vi "Seguidor Top Level.vi"() -> ()   [LabVIEW 2017]
uses:
  <vilib>/myRIO/Instrument Drivers/Onboard IO/I2C/typedefs/I2C User Configuration.ctl
  <vilib>/myRIO/Instrument Drivers/Onboard IO/I2C/typedefs/I2C Transfer Rate.ctl
  <vilib>/myRIO/Common/Instrument Driver Framework/myRIO v1.0/UART/vis/myRIO v1.0 Close UART.vi
  <vilib>/Utility/error.llb/Error Cluster From Error Code.vi
  <vilib>/myRIO/Common/Instrument Driver Framework/myRIO v1.0/I2C/vis/myRIO v1.0 Configure I2C.vi
  <vilib>/myRIO/Common/Instrument Driver Framework/Utilities/vis/FPGA Ref Manager.vi
  <vilib>/myRIO/Common/Instrument Driver Framework/myRIO v1.0/myRIO v1.0 Reset FPGA.vi
  <vilib>/myRIO/Common/Instrument Driver Framework/myRIO v1.0/IRQ/vis/myRIO v1.0 IRQ Info FGV.vi
  <vilib>/myRIO/Common/Instrument Driver Framework/myRIO v1.0/IRQ/vis/myRIO v1.0 Timer IRQ Info FGV.vi
  <vilib>/myRIO/Common/Instrument Driver Framework/myRIO v1.0/IRQ/vis/myRIO v1.0 ISR Agent.vi
  <vilib>/myRIO/Instrument Drivers/Onboard IO/I2C/I2C.lvlib
  <vilib>/myRIO/Instrument Drivers/Utilities/Utilities.lvlib
panel:
  in  "Boolean":bool
  in  "Enum":T1(ring)
  in  "stop":bool
  in  "Adelante/Atras":bool
  in  "Motor2":enum16{"MotorB", "MotorA"}(ring)
  in  "Motor1":enum16{"MotorB", "MotorA"}(ring)
  out "White":u8
  in  "Offset":dbl
  in  "Potencia \nmotores (%)":dbl(slide) scale=-100.0..100.0
  in  "Constante de \nProporcionalidad":dbl
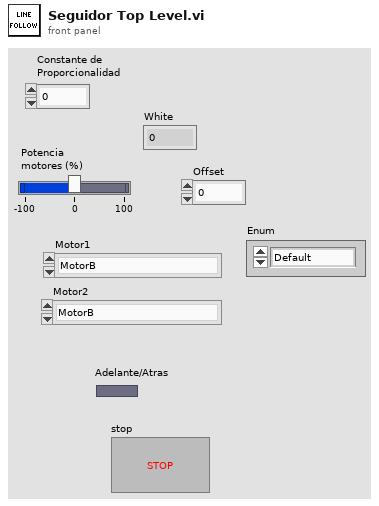
[diagram p1: front panel]
types:
  T1 = enum16{"Default", "Intersection", "Degrees", "Vision"}
  T2 = typedef "I2C.lvlib/I2C User Configuration.ctl" = cluster{"I2C Transfer Rate":T3}
  T3 = typedef "I2C.lvlib/I2C Transfer Rate.ctl" = enum16{"Standard mode (100 kbps)", "Fast mode (400 kbps)"}
  T4 = typedef "I2C.lvlib/I2C Reference.ctl" = cluster{"myRIO Reference":T5, "I2C Channels Enum":T9, "I2C Configuration":T10}
  T5 = typedef "myRIO Generic Hardware Reference.ctl" = cluster{"myRIO Model":T6, "myRIO Hardware Reference":T7}
  T6 = typedef "Hardware Version Enum.ctl" = enum16{"Unknown", "myRIO-1900", "myRIO-1950", "roboRIO", "NI ELVIS RIO CM"}
  T7 = typedef "myRIO v1.0 Reference.ctl" = cluster{"Generic FPGA Reference":T8, "Allow multiple opens":bool}
  T8 = typedef "Generic FPGA Reference.ctl" = refnum<k20>
  T9 = typedef "I2C Channels Enum.ctl" = enum16{"Not Connected", "A/I2C", "B/I2C", "I2C/I2C"}
  T10 = typedef "I2C.lvlib/I2C Configuration.ctl" = cluster{"I2C Transfer Rate":T3}
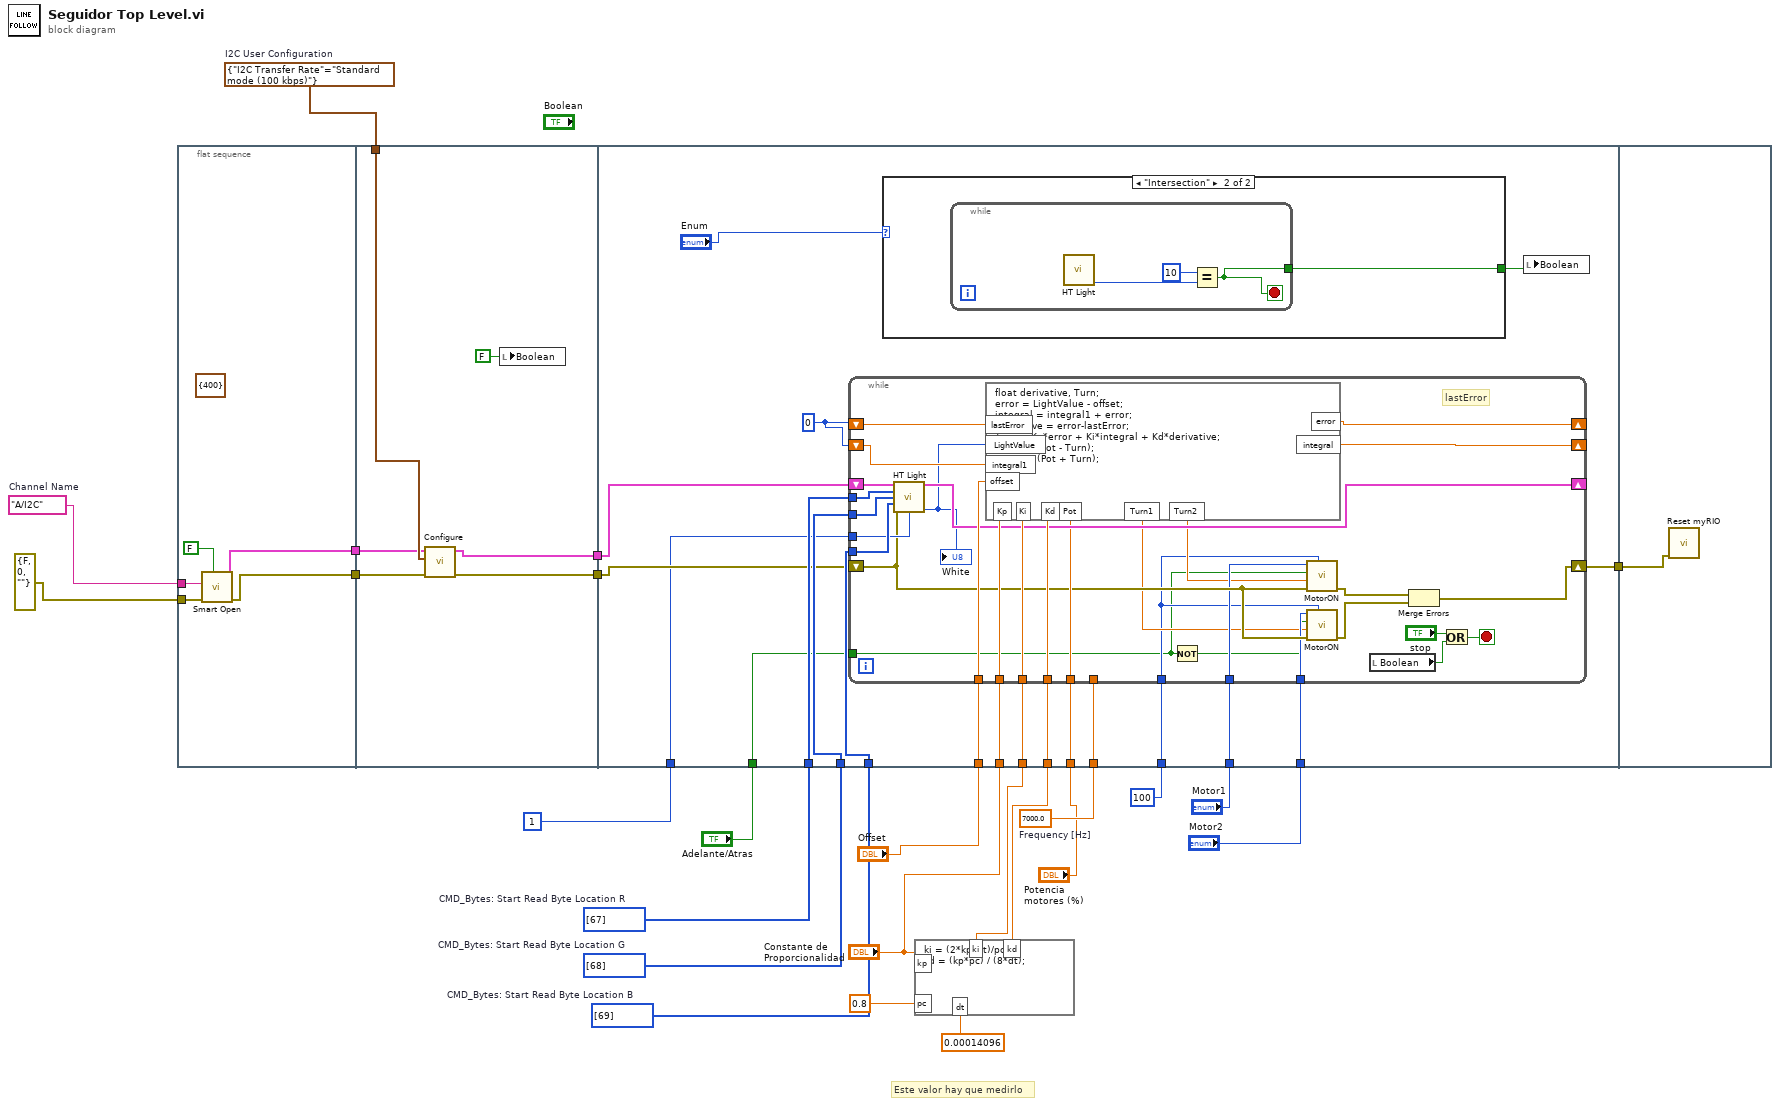
[diagram p0: block diagram]
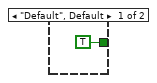
[diagram p2: hidden frame]
diagram:
  w10 = T2 {"I2C Transfer Rate"=enum."Standard mode (100 kbps)"}  # I2C User Configuration
  w12 = tag "A/I2C"  # Channel Name
  w15 = 7000.0  # Frequency [Hz]
  w22 = u8[] [69]  # CMD_Bytes: Start Read Byte Location B
  w23 = u8[] [68]  # CMD_Bytes: Start Read Byte Location G
  w24 = u8[] [67]  # CMD_Bytes: Start Read Byte Location R
  # "Este valor hay que medirlo"
  n1 = flat-sequence {
    tunnel: errorcluster {"status"=FALSE, "code"=0, "source"=""} ("error in (no error)") -> [w29]
    tunnel: w12 -> [w28]
    tunnel: [w26] -> w11
    tunnel: [w25] -> w9
    tunnel: w11 -> [w35]
    tunnel: w10 -> [w34]
    tunnel: w9 -> [w33]
    tunnel: [w32] -> w8
    tunnel: [w31] -> w7
    tunnel: w24 -> [w55]
    tunnel: w23 -> [w54]
    tunnel: w22 -> [w53]
    tunnel: w19 -> [w52]
    tunnel: w18 -> [w51]
    tunnel: "Constante de \nProporcionalidad" -> [w50]
    tunnel: "Offset" -> [w48]
    tunnel: w15 -> [w47]
    tunnel: "Potencia \nmotores (%)" -> [w46]
    tunnel: w8 -> [w44]
    tunnel: w7 -> [w45]
    tunnel: u8 1 -> [w43]
    tunnel: [w42] -> w5
    tunnel: "Motor1" -> [w41]
    tunnel: "Motor2" -> [w40]
    tunnel: 100 -> [w39]
    tunnel: "Adelante/Atras" -> [w38]
    tunnel: w5 -> [w91]
    frame #0 {
      (unwired) cluster{"SCL Period (Ticks)":u32} {"SCL Period (Ticks)"=400} ("Protocol_Timing")
      n2 = call <vilib>:"Smart Open.vi"("Allow multiple opens?"=FALSE, "error in (no error)"=w29, "Channel Name"=w28) -> ("error out"=w26:errorcluster, "I2C Ref Out"=w25:T4)  [unwired: 7 in]
    }
    frame #1 {
      n3 = call <vilib>:"Configure.vi"("error in (no error)"=w35, "I2C User Configuration"=w34, "I2C Ref In"=w33) -> ("error out"=w31:errorcluster, "I2C Ref Out"=w32:T4)  [unwired: 7 in]
      n4 = local write "Boolean"(FALSE ("Boolean")) -> ()
    }
    frame #2 {
      w49 = 0
      n5 = while {
        tunnel: w55 -> [w79]
        tunnel: w54 -> [w78]
        tunnel: w53 -> [w77]
        shift-right: [w85] -> _
        shift-left: w49 -> [w86]
        tunnel: w52 -> [w87]
        tunnel: w51 -> [w88]
        tunnel: w50 -> [w89]
        shift-right: [w84] -> _
        shift-left: w49 -> [w83]
        tunnel: w48 -> [w82]
        tunnel: w47 -> [_]
        tunnel: w46 -> [w80]
        tunnel: w43 -> [w76]
        shift-right: [w74] -> w42
        shift-left: w45 -> [w73]
        shift-right: [w81] -> _
        shift-left: w44 -> [w90]
        tunnel: w41 -> [w70]
        tunnel: w40 -> [w69]
        tunnel: w39 -> [w66]
        tunnel: w38 -> [w64]
        stop <- w61 stop-if-true
        # "lastError"
        n6 = call "HT Light.vi"("I2C Ref In"=w90, "Data Red"=w79, "Data Green"=w78, "Data Blue"=w77, "error in (no error)"=w73, "Address"=w76) -> ("I2C Ref Out"=w81:T4, "White"=w75:u8)  [unwired: 4 in, 4 out]
        "White" <- w75
        n7 = formula code="float derivative, Turn;\nerror = LightValue - offset;\nintegral = integral1 + error; \nderivative = error-lastError;\nTurn = Kp*error + Ki*integral + Kd*derivative;\nTurn1 = (Pot - Turn);\nTurn2 = (Pot + Turn);"("LightValue"=w75, "Kp"=w89, "Ki"=w87, "Kd"=w88, "lastError"=w86, "integral1"=w83, "offset"=w82, "Pot"=w80) -> ("error"=w85:dbl, "integral"=w84:dbl, "Turn1"=w68:dbl, "Turn2"=w67:dbl)
        n8 = Not(x=w64) -> (.not. x?=w65:bool)
        n9 = call "MotorON.vi"("y"=w66, "error in (no error)"=w73, "Power (%)"=w67, "(Antihorario) Direction (Horario)"=w64, "Enum"=w70) -> ("error out"=w71:errorcluster)  [unwired: 6 in]
        n10 = call "MotorON.vi"("y"=w66, "error in (no error)"=w73, "Power (%)"=w68, "(Antihorario) Direction (Horario)"=w65, "Enum"=w69) -> ("error out"=w72:errorcluster)  [unwired: 6 in]
        n11 = local read "Boolean"() -> (w63:bool)
        n12 = Merge Errors(w71, w72) -> (w74:errorcluster)
        n13 = Or(x="stop", y=w63) -> (x .or. y?=w61:bool)
      }
      n14 = case shown="\"Intersection\"" "Enum" {
        tunnel: [TRUE w57] -> w36
        frame "Default", Default {
        }
        frame "Intersection" {
          n15 = while {
            tunnel: [w58] -> w57
            stop <- w58 stop-if-true
            n16 = call "HT Light.vi"() -> ("White"=w60:u8)  [unwired: 10 in, 5 out]
            n17 = Equal?(x=u8 10, y=w60) -> (x = y?=w58:bool)
          }
        }
      }
      n18 = local write "Boolean"(w36) -> ()
    }
    frame #3 {
      n19 = call <vilib>:"Reset myRIO.vi"("error in (no error)"=w91) -> ()  [unwired: 10 in, 1 out]
    }
  }
  n20 = formula code="ki = (2*kp*dt)/pc;\nkd = (kp*pc) / (8*dt);"("kp"="Constante de \nProporcionalidad", "dt"=0.00014096, "pc"=0.8) -> ("ki"=w19:dbl, "kd"=w18:dbl)
